vi "Algorithms.vi"() -> ()   [LabVIEW 2013]
uses:
  qwtblvlib/TD Algorithm Information.ctl
  qwtblvlib/TD Algorithm Information Input.ctl
  qwtblvlib/TD Algorithm Information Output.ctl
  globals.vi
  qwtblvlib/QWTBLVLib.lvlib
panel:
  in  "curAlg":u16(ring) caption="Selected Algorithm ID" items=["4PSWF", "ADEV", "FourPSF", "INL-DNL", "MADEV", "OADEV", "PSFE", "SFDR", "SINAD-ENOB", "SP-FFT", "ThreePSF", "iDFT2p", "iDFT3p", "testG", "testGM", "testM", "testQ"]
  out "Algorithm Information":T1
  in  "reload alginfo":bool
  in  "close":bool
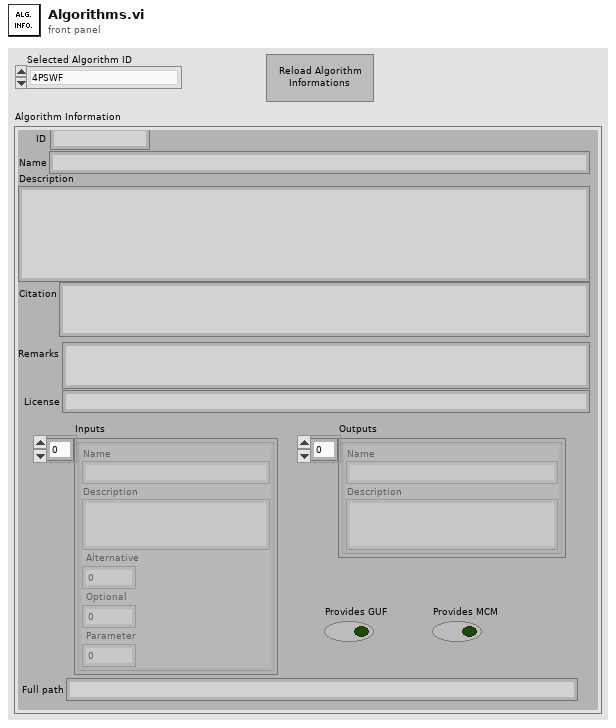
[diagram p1: front panel]
types:
  T1 = typedef "QWTBLVLib.lvlib/TD Algorithm Information.ctl" = cluster{"ID":string, "Name":string, "Description":string, "Citation":string, "Remarks":string, "License":string, "Inputs":T2[], "Outputs":T3[], "Provides GUF":bool, "Provides MCM":bool, "Full path":string}
  T2 = typedef "QWTBLVLib.lvlib/TD Algorithm Information Input.ctl" = cluster{"Name":string, "Description":string, "Alternative":i32, "Optional":i32, "Parameter":i32}
  T3 = typedef "QWTBLVLib.lvlib/TD Algorithm Information Output.ctl" = cluster{"Name":string, "Description":string}
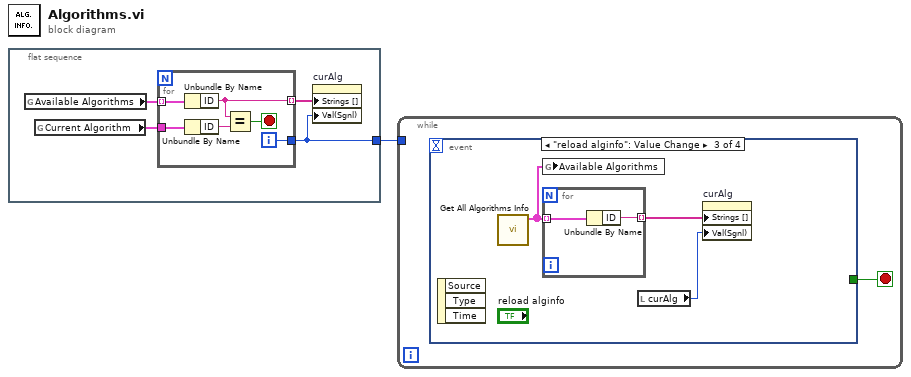
[diagram p0: block diagram]
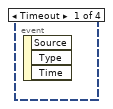
[diagram p2: hidden frame]
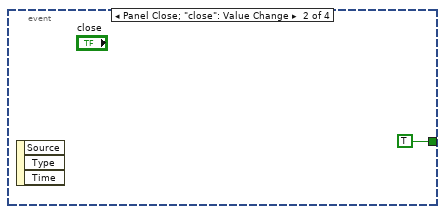
[diagram p3: hidden frame]
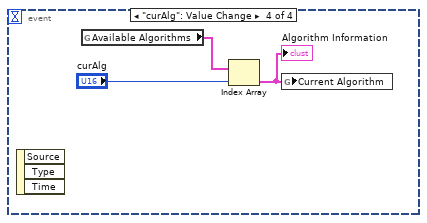
[diagram p4: hidden frame]
diagram:
  n1 = flat-sequence {
    tunnel: [w3] -> w1
    frame #0 {
      n2 = global read "globals.vi" "Available Algorithms"() -> (w4:T1[])
      n3 = global read "globals.vi" "Current Algorithm"() -> (w5:T1)
      n4 = for {
        tunnel: w5 -> [w10]
        tunnel: w4 -> [w11] mode=indexing
        tunnel: [w7] -> w3
        tunnel: [w6] -> w2 mode=indexing
        i -> [w7]
        stop <- w8 stop-if-true
        n5 = Unbundle By Name(w11) -> ("ID"=w6:string)
        n6 = Unbundle By Name(w10) -> ("ID"=w9:string)
        n7 = Equal?(x=w6, y=w9) -> (x = y?=w8:bool)
      }
      n8 = property on="curAlg" class="Ring (strict)"("Strings []"=w2, "Val(Sgnl)"=w3) -> ()  [unwired: 2 in, 2 out]
    }
  }
  n9 = while {
    tunnel: w1 -> [_]
    stop <- w12 stop-if-true
    n10 = event shown="[2] \"reload alginfo\": Value Change" {
      selector: _ -> [_ _ _ _]
      dyn-events: _ -> [_ _ _ _]
      timeout: _ -> [_ _ _ _]
      tunnel: [_ TRUE ("cancel") _ _] -> w12
      event Timeout {
        n11 = event-data() -> ()  [unwired: 1 in, 3 out]
      }
      event Panel Close; "close": Value Change {
        n12 = event-data() -> ()  [unwired: 1 in, 3 out]
      }
      event "reload alginfo": Value Change {
        n13 = event-data() -> ()  [unwired: 1 in, 3 out]
        n14 = call "Get All Algorithms Info.vi"() -> ("All Algorithms Info"=w16:T1[])  [unwired: 10 in, 1 out]
        n15 = global write "globals.vi" "Available Algorithms"(w16) -> ()
        n16 = for {
          tunnel: w16 -> [w18] mode=indexing
          tunnel: [w17] -> w14 mode=indexing
          n17 = Unbundle By Name(w18) -> ("ID"=w17:string)
        }
        n18 = local read "curAlg"() -> (w15:u16)
        n19 = property on="curAlg" class="Ring (strict)"("Strings []"=w14, "Val(Sgnl)"=w15) -> ()  [unwired: 2 in, 2 out]
      }
      event "curAlg": Value Change {
        n20 = event-data() -> ()  [unwired: 1 in, 3 out]
        n21 = global read "globals.vi" "Available Algorithms"() -> (w21:T1[])
        n22 = Index Array(array=w21, index="curAlg") -> (element=w19:T1)
        "Algorithm Information" <- w19
        n23 = global write "globals.vi" "Current Algorithm"(w19) -> ()
      }
    }
  }
